vi "Equality Check Set and Response.vi"(8 "error in (no error)":errorcluster, 10 "Sent":string, 11 "Response":string) -> (0 "error out":errorcluster)   [LabVIEW 2023, in "OWON SDS1022.lvlib" / "SDS1000 Base CFG.lvclass"]
uses:
  SDS1000 Base CFG.lvclass
  SDS1000 Base CFG.lvclass/SDS1000 Base CFG.ctl
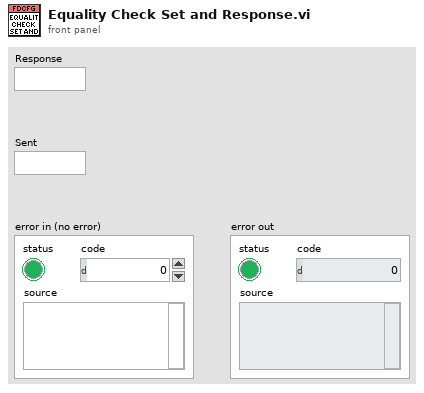
[diagram p1: front panel]
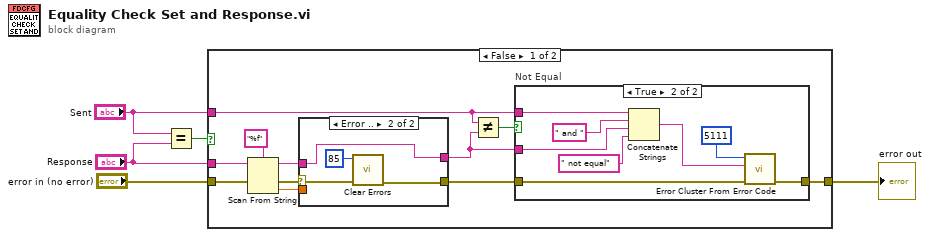
[diagram p0: block diagram]
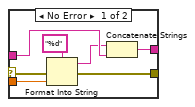
[diagram p2: hidden frame]
diagram:
  n1 = Equal?(x="Sent", y="Response") -> (x = y?=w2:bool)
  n2 = case shown="False" w2 {
    tunnel: "error in (no error)" -> [w14 w37]
    tunnel: [w9 w37] -> w4
    tunnel: "Sent" -> [w7 _]
    tunnel: "Response" -> [w6 _]
    frame False {
      n3 = Scan From String(format string="%f", input string=w6, error in=w14) -> (remaining string=w15:string, error out=w11:errorcluster, output 1=w12:dbl)  [unwired: 2 in, 1 out]
      n4 = case shown="Error .." w11 {
        selector: w11 -> [w23 w27]
        tunnel: w12 -> [w21 _]
        tunnel: [w22 w26] -> w13
        tunnel: w15 -> [w19 w24]
        tunnel: [w17 w24] -> w16
        frame No Error {
          n5 = Format Into String(format string="%d", error in=w23, w21) -> (resulting string=w18:string, error out=w22:errorcluster)  [unwired: 1 in]
          n6 = Concatenate Strings(w18, w19) -> (w17:string)
        }
        frame Error {
          n7 = call <vilib>:"Clear Errors.vi"("error in (no error)"=w27, "specific error code to clear (0: all)"=85) -> ("error out"=w26:errorcluster)  [unwired: 4 in, 1 out]
        }
      }
      n8 = Not Equal?(x=w7, y=w16) -> (x != y?=w8:bool)
      n9 = case "Not Equal" shown="True" w8 {
        tunnel: w13 -> [w28 w36]
        tunnel: [w28 w35] -> w9
        tunnel: w7 -> [_ w34]
        tunnel: w16 -> [_ w32]
        frame False {
        }
        frame True {
          n10 = Concatenate Strings(w34, " and " ("string"), w32, " not equal" ("string")) -> (w30:string)
          n11 = call <vilib>:"Error Cluster From Error Code.vi"("error in (no error)"=w36, "error message (\"\")"=w30, "error code (0)"=5111) -> ("error out"=w35:errorcluster)  [unwired: 6 in]
        }
      }
    }
    frame True {
    }
  }
  "error out" <- w4
